vi "Check 985x DMA.vi"(8 "error in (no error)":errorcluster, 11 "Bitfile path":path=path "\\\\vmware-host\\Shared Folders/_Repo/CAN-Frame-Protection-Custom-Device/Source/SubModules/985x-Support/Source/FPGA Bitfiles/985xsupport_FPGATarget_fpga-main_5XgmTEdlmQU.lvbitx") -> (0 "error out":errorcluster, 2 "Available Channels":string[](array[string]), 3 "Found":bool)   [LabVIEW 2020, in "985x Support System Explorer.lvlib"]
uses:
  985x Support System Explorer.lvlib
  <vilib>/rvi/ClientSDK/Host Interface/DMA/public/niFpgaDmaChannelVisibilityFilter.ctl
  <vilib>/rvi/ClientSDK/Core/ModuleGeneration/CommunicationInterfaceUtility/niFpgaDmaChannelImplementation.ctl
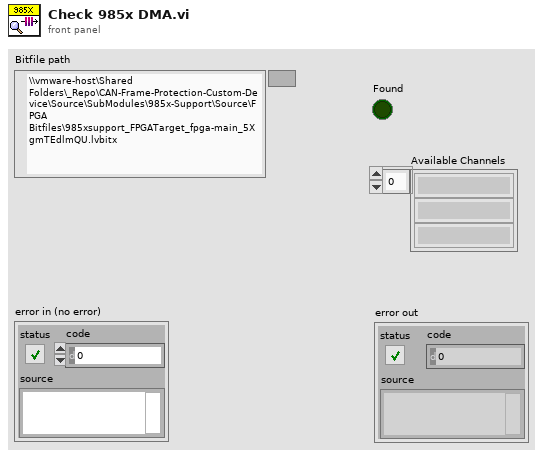
[diagram p1: front panel]
types:
  T1 = typedef "niFpgaDmaChannelVisibilityFilter.ctl" = enum16{"All", "UserVisible"}
  T2 = typedef "niFpgaDmaChannelImplementation.ctl" = enum16{"niFpgaTargetToHost", "niFpgaHostToTarget", "niFpgaPeerToPeerWriter", "niFpgaPeerToPeerReader", "niCoreTargetToHost", "niCoreHostToTarget"}
  T3 = typedef "Fifo_DMA_Config.ctl" = cluster{"Name":string, "Depth":u32, "Write? (Deprecated:Use Implementation)":bool, "Physical Channel":u32, "Base Address":u32, "Data Width":u32, "Data Type":T4, "FXP Properties":variant, "Write Window Address":u32, "Implementation":T2, "Control Set":u32}
  T4 = typedef "niFpgaDataTypeControl.ctl" = enum32{"Boolean", "I8", "I16", "I32", "I64", "U8", "U16", "U32", "U64", "FXP", "CustomControl", "SGL"}
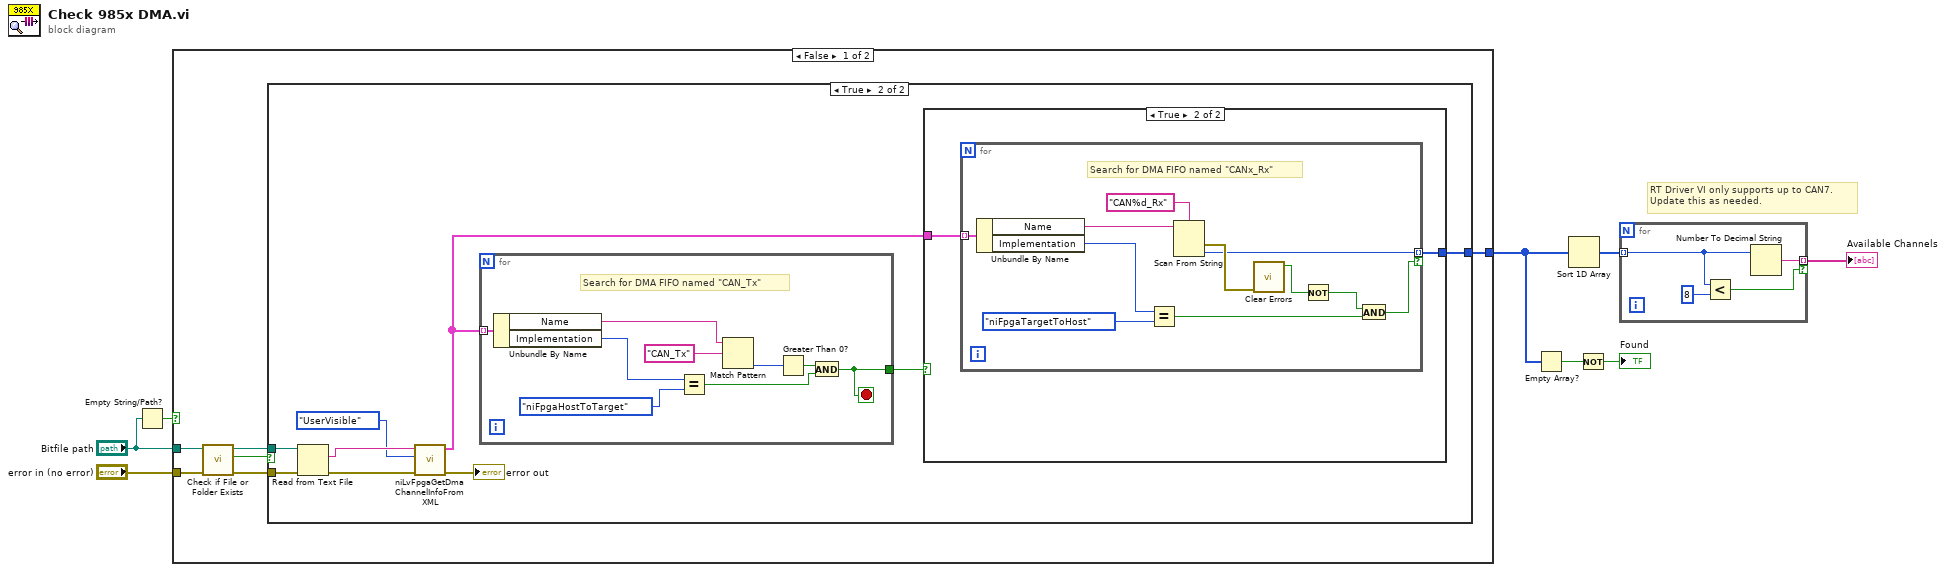
[diagram p0: block diagram]
diagram:
  # "RT Driver VI only supports up to CAN7. \nUpdate this as needed."
  n1 = Empty String/Path?(string/path="Bitfile path") -> (empty?=w1:bool)
  n2 = case shown="False" w1 {
    tunnel: "error in (no error)" -> [w14 _]
    tunnel: [w10 _] -> w4
    tunnel: "Bitfile path" -> [w9 _]
    frame False {
      n3 = call <vilib>:"Check if File or Folder Exists.vi"("error in (no error)"=w14, "path"=w9) -> ("error out"=w13:errorcluster, "file or folder exists?"=w11:bool, "dup path"=w12:path)  [unwired: 7 in]
      n4 = case shown="True" w11 {
        tunnel: w12 -> [_ w23]
        tunnel: w13 -> [_ w22]
        tunnel: [_ w15] -> w10
        frame False {
        }
        frame True {
          n5 = Read from Text File(file (use dialog)=w23, error in=w22) -> (text=w21:string, error out=w20:errorcluster)  [unwired: 2 in, 2 out]
          n6 = call <resource>:"niLvFpgaGetDmaChannelInfoFromXML.vi"("error in (no error)"=w20, "DMA Channel Filter"=niFpgaDmaChannelVisibilityFilter."UserVisible", "XML String in"=w21) -> ("error out"=→"error out":errorcluster, "DMA configuration array"=w17:T3[])  [unwired: 7 in]
          n7 = for {
            tunnel: w17 -> [w32] mode=indexing
            tunnel: [w24] -> w16
            stop <- w24 stop-if-true
            # "Search for DMA FIFO named \"CAN_Tx\""
            n8 = Unbundle By Name(w32) -> ("Name"=w25:string, "Implementation"=w26:T2)
            n9 = Equal?(x=w26, y=niFpgaDmaChannelImplementation."niFpgaHostToTarget" ("Implementation")) -> (x = y?=w27:bool)
            n10 = Match Pattern(string=w25, regular expression="CAN_Tx") -> (offset past match=w29:i32)  [unwired: 1 in, 3 out]
            n11 = Greater Than 0?(x=w29) -> (x > 0?=w28:bool)
            n12 = And(x=w28, y=w27) -> (x .and. y?=w24:bool)
          }
          n13 = case shown="True" w16 {
            tunnel: w17 -> [_ w34]
            tunnel: [_ w33] -> w15
            frame False {
            }
            frame True {
              n14 = for {
                tunnel: w34 -> [w45] mode=indexing
                tunnel: [w36] -> w33 mode=indexing if=w35
                # "Search for DMA FIFO named \"CANx_Rx\""
                n15 = Unbundle By Name(w45) -> ("Name"=w41:string, "Implementation"=w43:T2)
                n16 = Equal?(x=w43, y=niFpgaDmaChannelImplementation."niFpgaTargetToHost" ("Implementation")) -> (x = y?=w37:bool)
                n17 = Scan From String(format string="CAN%d_Rx" ("regular expression"), input string=w41) -> (error out=w40:errorcluster, output 1=w36:i32)  [unwired: 3 in, 2 out]
                n18 = call <vilib>:"Clear Errors.vi"("error in (no error)"=w40) -> ("specific error cleared?"=w39:bool)  [unwired: 5 in, 1 out]
                n19 = Not(x=w39) -> (.not. x?=w38:bool)
                n20 = And(x=w38, y=w37) -> (x .and. y?=w35:bool)
              }
            }
          }
        }
      }
    }
    frame True {
    }
  }
  n21 = Empty Array?(array=w4) -> (empty?=w7:bool)
  n22 = Sort 1D Array(array=w4) -> (sorted array=w3:i32[])
  n23 = Not(x=w7) -> (.not. x?=→"Found":bool)
  n24 = for {
    tunnel: w3 -> [w48] mode=indexing
    tunnel: [w49] -> w5 mode=indexing if=w46
    n25 = Less?(x=w48, y=8) -> (x < y?=w46:bool)
    n26 = Number To Decimal String(number=w48) -> (decimal integer string=w49:string)  [unwired: 1 in]
  }
  "Available Channels" <- w5
